vi "TDMS Upload.vi"(0 "Sift Client in":refnum<class "Sift Client.lvclass">, 1 "run_id":string, 5 "filepath":string, 7 "asset_name":string, 9 "group_into_components":bool, 11 "error in (no error)":errorcluster, 12 "run_name":string, 13 "timeout":i32=-1) -> (4 "Sift Client out":refnum<class "Sift Client.lvclass">, 15 "error out":errorcluster)   [LabVIEW 2024, in "Sift Client.lvlib" / "Sift Client.lvclass"]
uses:
  Sift Client.lvclass
  Sift Client.lvclass/Sift Client.ctl
  Sift Client.lvlib
  <vilib>/addons/_JKI.lib/Serialization/JSON/JKI JSON Serialization.lvlib
  Private/Typedefs/Messages/JSON Request.ctl
  Private/Typedefs/Messages/TDMS Upload Request.ctl
panel:
  in  "TDMS Upload Request":T1
  in  "JSON Request":T2
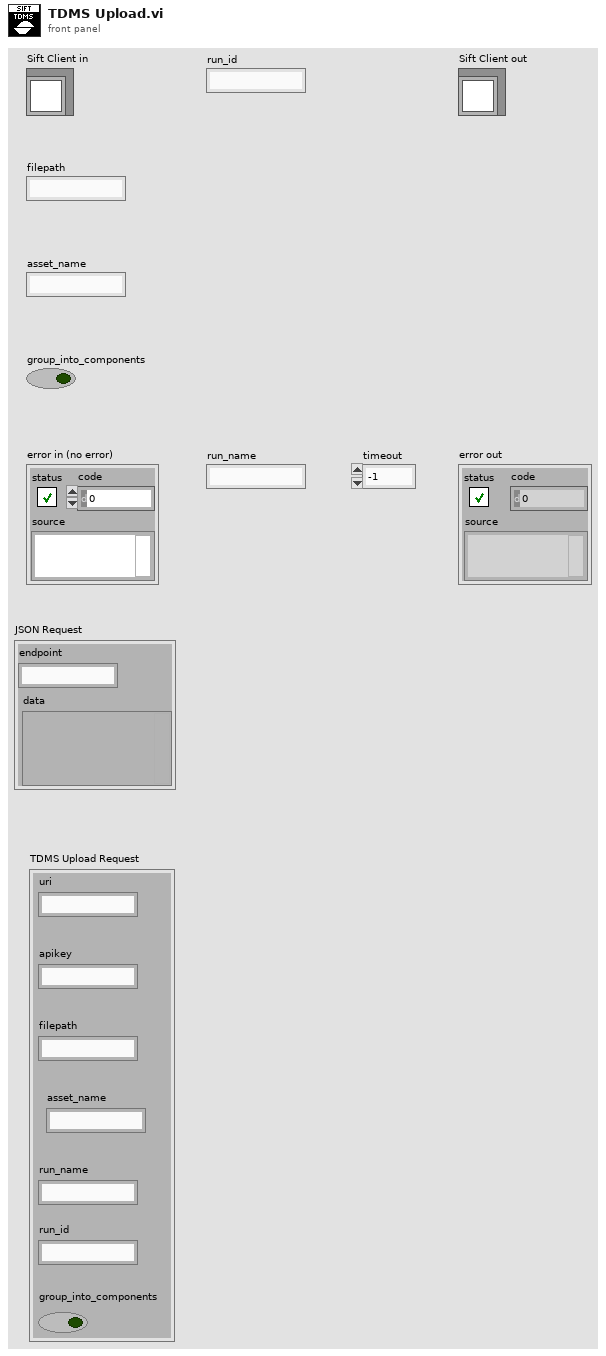
[diagram p1: front panel]
types:
  T1 = typedef "Sift Client.lvlib/TDMS Upload Request.ctl" = cluster{"uri":string, "apikey":string, "filepath":string, "asset_name":string, "run_name":string, "run_id":string, "group_into_components":bool}
  T2 = typedef "Sift Client.lvlib/JSON Request.ctl" = cluster{"endpoint":string, "data":variant}
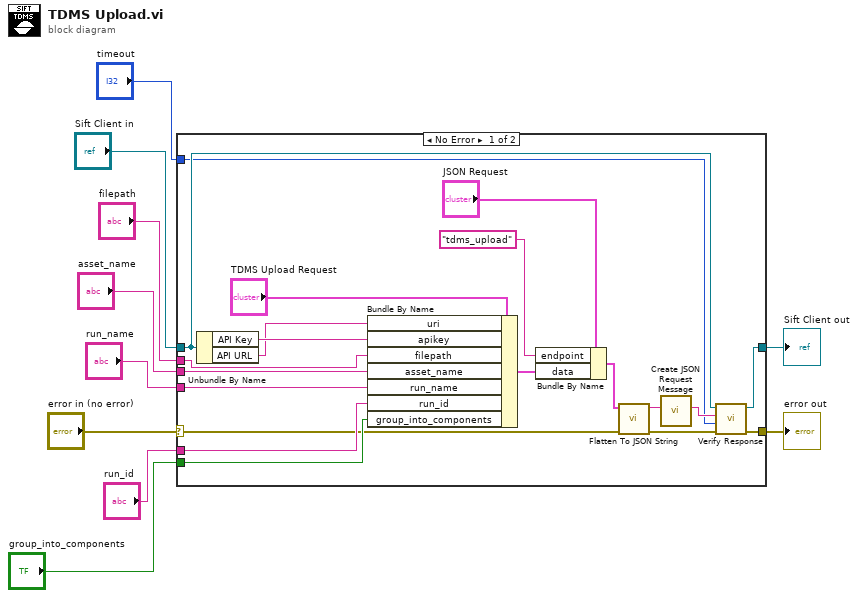
[diagram p0: block diagram]
diagram:
  n1 = case shown="No Error" "error in (no error)" {
    selector: "error in (no error)" -> [w14 w32]
    tunnel: [w12 w32] -> w9
    tunnel: [w15 w31] -> w7
    tunnel: "Sift Client in" -> [w16 w31]
    tunnel: "filepath" -> [w29 _]
    tunnel: "asset_name" -> [w28 _]
    tunnel: "run_name" -> [w27 _]
    tunnel: "run_id" -> [w26 _]
    tunnel: "group_into_components" -> [w25 _]
    tunnel: "timeout" -> [w11 _]
    frame No Error {
      n2 = Unbundle By Name(w16) -> ("API Key"=w24:string, "API URL"=w23:string)
      n3 = Bundle By Name(cluster="TDMS Upload Request", "uri"=w23, "apikey"=w24, "filepath"=w29, "asset_name"=w28, "run_name"=w27, "run_id"=w26, "group_into_components"=w25) -> (w21:T1)
      n4 = Bundle By Name(cluster="JSON Request", "endpoint"="tdms_upload", "data"=w21) -> (w19:T2)
      n5 = call <vilib>:"Flatten To JSON String.vi"("error in"=w14, "Variant"=w19) -> ("error out"=w13:errorcluster, "JSON String"=w18:string)  [unwired: 8 in]
      n6 = call "Create JSON Request Message.vi"("Data"=w18) -> ("Message"=w17:string)  [unwired: 10 in]
      n7 = call-dynamic "Verify Response.vi"("error in (no error)"=w13, "timeout ms (25000)"=w11, "Message"=w17, "Sift Client in"=w16) -> ("error out"=w12:errorcluster, "Sift Client out"=w15:refnum<class "Sift Client.lvclass">)  [unwired: 5 in, 1 out]
    }
    frame Error {
    }
  }
  "error out" <- w9
  "Sift Client out" <- w7
